vi "Device_Connect.vi"() -> ()   [LabVIEW 2020]
uses:
  User_Manage/User_Databse/User String.ctl
  <vilib>/Retry/UI Control Suite/Boolean/System Buttons/Connect Button.ctl
  Driver/E5071C/E5071C/E5071C.lvclass
  Driver/PEU/PEU/PEU.lvclass
  <vilib>/Utility/cursorutil.llb/Set Cursor (Icon Pict).vi
panel:
  in  "Title":string="设备连接"
  out "User Info":T1
  in  "Connect_PEU":T2
  in  "Port_PEU":u16=4001 caption="Port:"
  in  "IP_PEU":string="192.167.1.11" caption="IP Address:"
  out "Device_PEU":string caption="Device:"
  in  "Next Button":bool
  in  "Connect_E5071C":T2
  in  "Port_ENA":u16 caption="Port:"
  in  "IP_ENA":string="192.167.1.100" caption="IP Address:"
  out "Device_ENA":string caption="Device:"
  out "Time String":string
  # "E5071C"
  # "PEU"
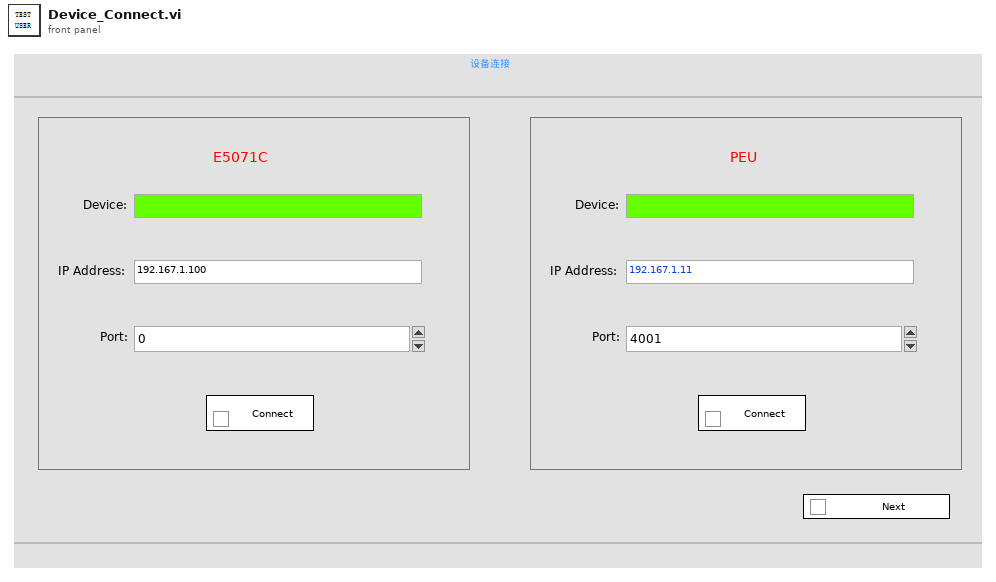
[diagram p1: front panel]
types:
  T1 = typedef "User String.ctl" = string
  T2 = typedef "Connect Button.ctl" = bool
  T3 = enum8{"Enabled", "Disabled", "Disabled and Grayed Out"}
  T4 = cluster{"User_Right":u16, "E5071C":refnum<class "E5071C.lvclass">, "PEU":refnum<class "PEU.lvclass">, "Next_OK":cluster{"ENA_OK":bool, "PEU_OK":bool}}
  T5 = typedef "User_Info.ctl" = cluster{"Name":string, "Password":string, "User_Right":u16, "Debuger?":bool, "Manager?":bool, "User_Remember_Name":bool, "User_Remember_PW":bool, "User_Right_String":string, "Null?":bool, "Language":string}
  T6 = enum32{"invalid app kind", "Development System", "Run Time System", "Student Edition", "Embedded LabVIEW", "Evaluation", "Custom"}
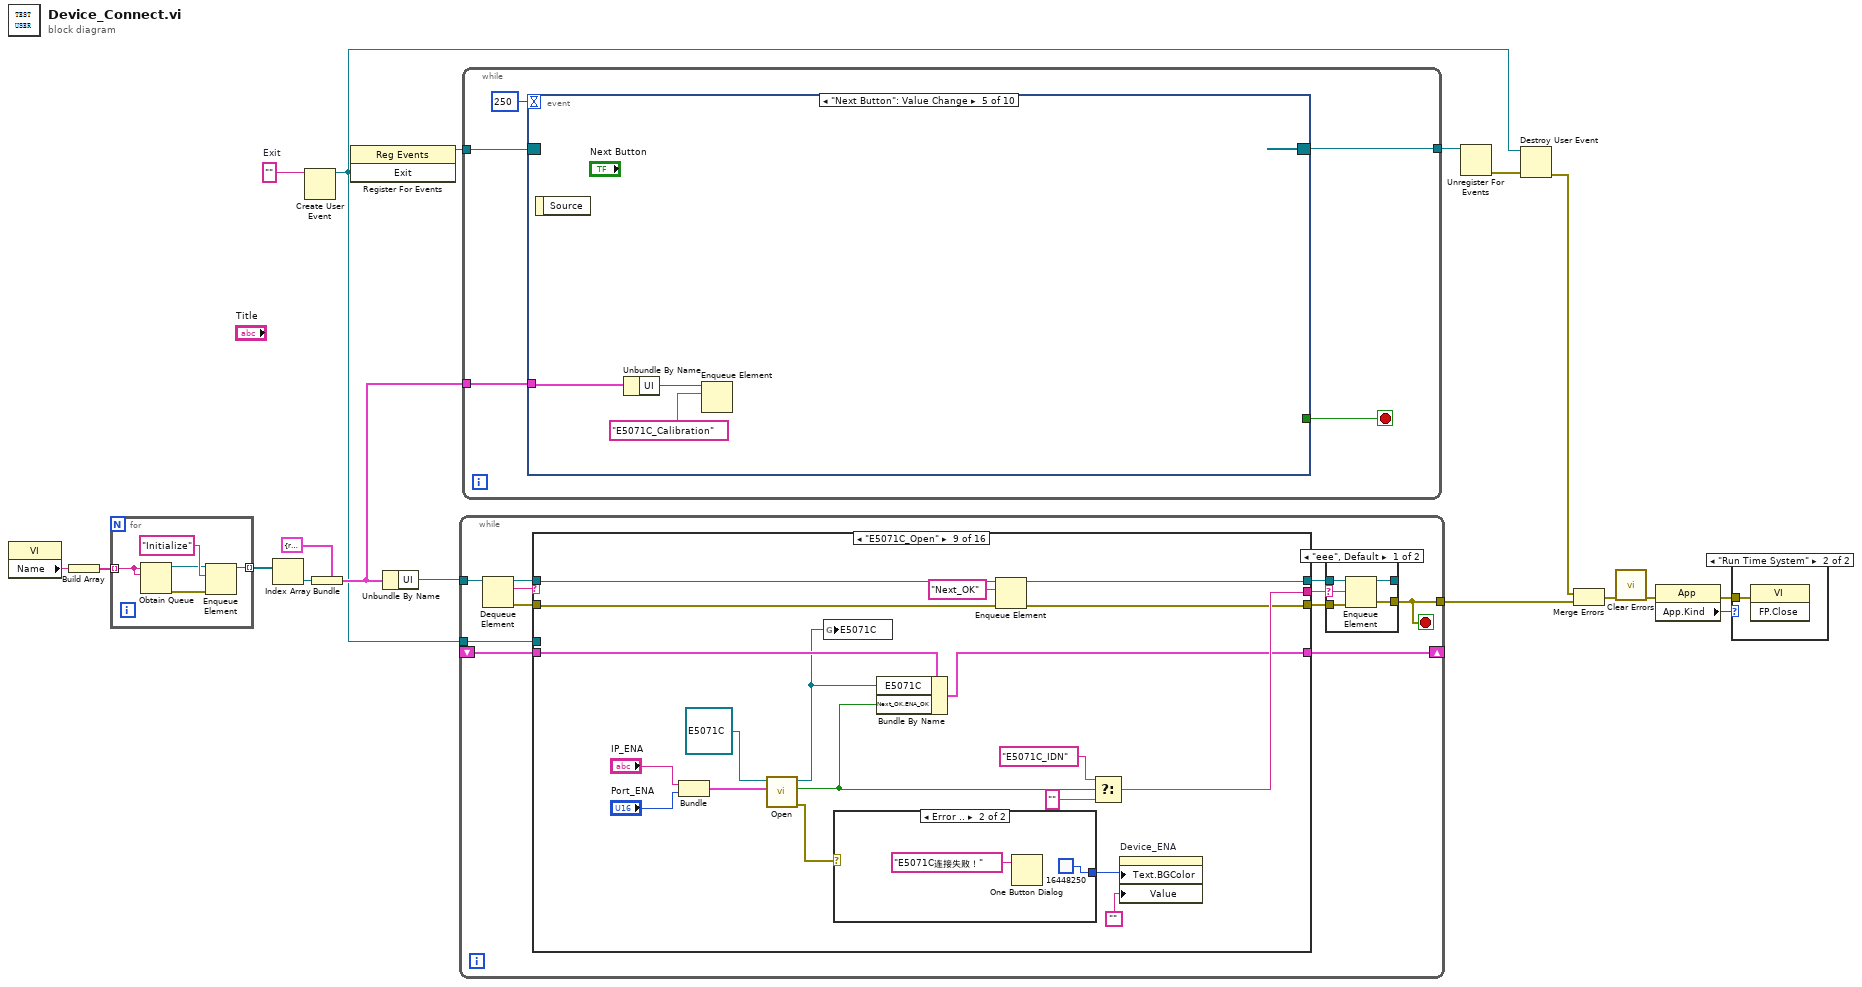
[diagram p0: block diagram]
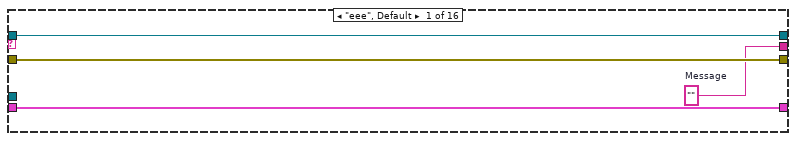
[diagram p4: hidden frame]
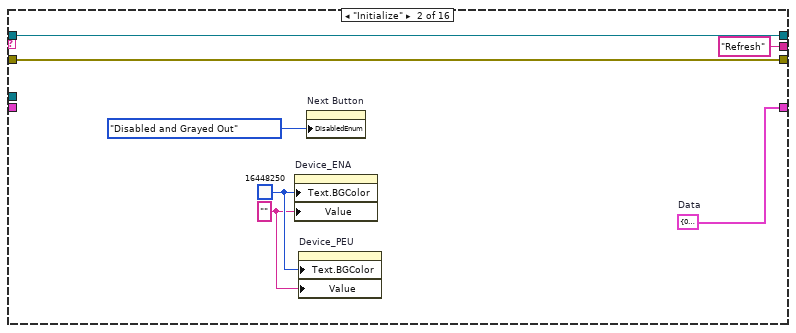
[diagram p5: hidden frame]
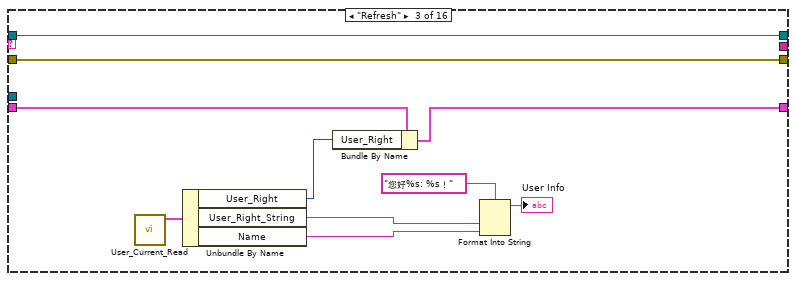
[diagram p6: hidden frame]
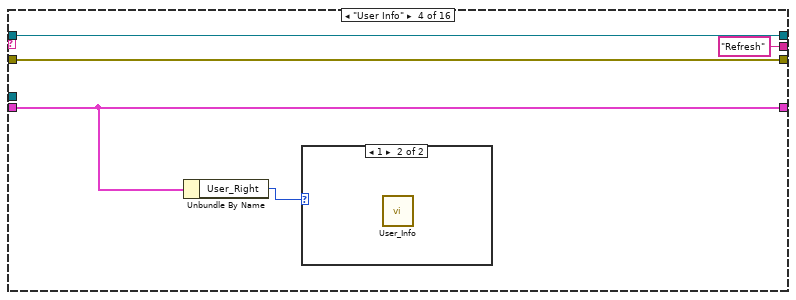
[diagram p7: hidden frame]
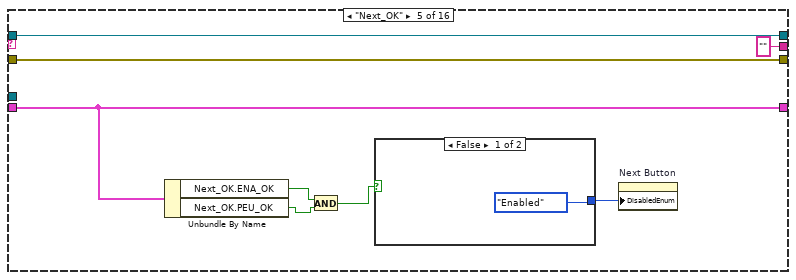
[diagram p9: hidden frame]
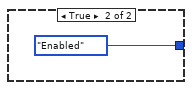
[diagram p10: hidden frame]
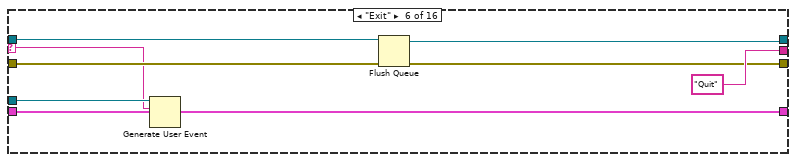
[diagram p11: hidden frame]
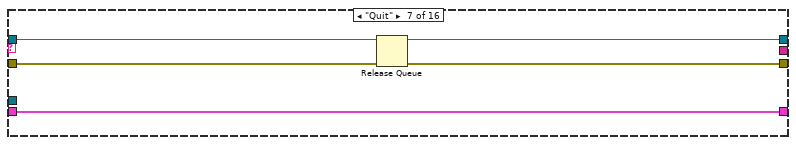
[diagram p12: hidden frame]
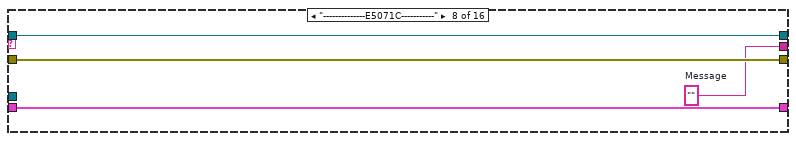
[diagram p13: hidden frame]
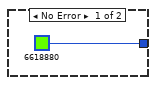
[diagram p14: hidden frame]
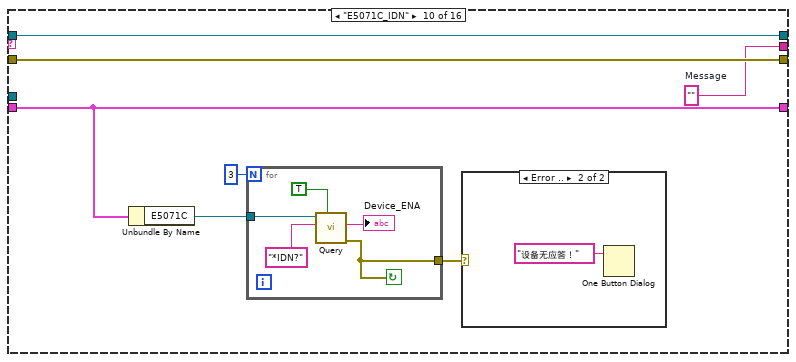
[diagram p15: hidden frame]
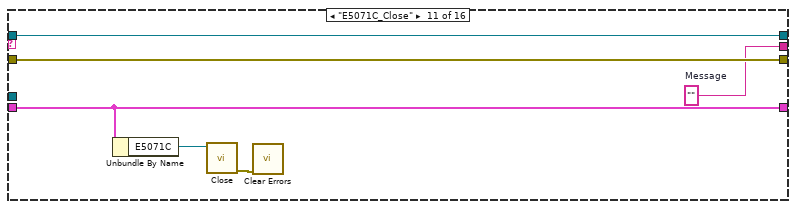
[diagram p17: hidden frame]
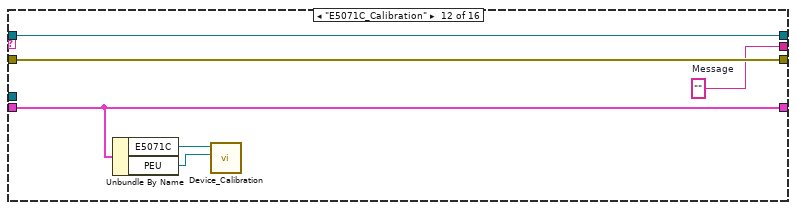
[diagram p18: hidden frame]
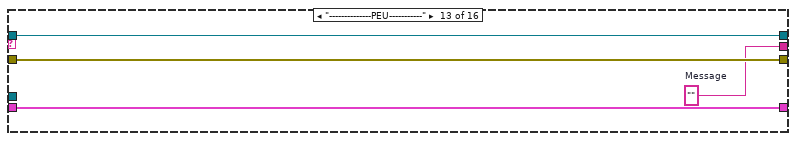
[diagram p19: hidden frame]
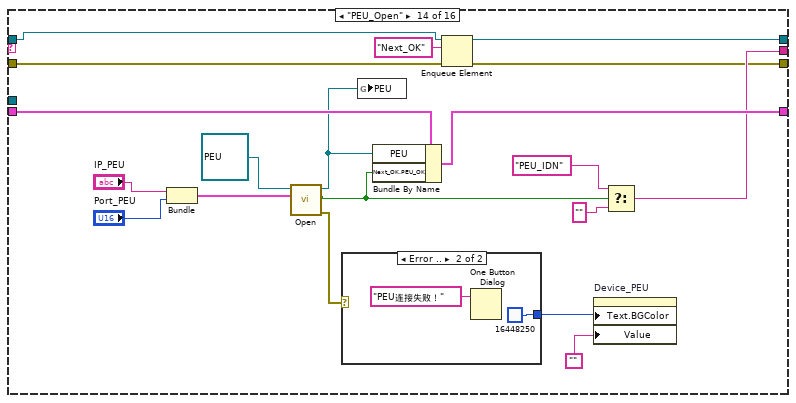
[diagram p20: hidden frame]
diagram:
  w3 = ""  # Exit
  n1 = property class="VI"() -> ("Name"=w13:string)  [unwired: 2 in, 2 out]
  n2 = Build Array(w13) -> (w14:string[])
  n3 = for {
    tunnel: w14 -> [w19] mode=indexing
    tunnel: [w20] -> w8 mode=indexing
    n4 = Obtain Queue(name (unnamed)=w19, element data type=w19) -> (queue out=w22:refnum<queue>, error out=w21:errorcluster)  [unwired: 3 in, 1 out]
    n5 = Enqueue Element(queue=w22, element="Initialize" ("元素"), error in (no error)=w21) -> (queue out=w20:refnum<queue>)  [unwired: 1 in, 2 out]
  }
  n6 = Index Array(array=w8) -> (element=w11:refnum<queue>)  [unwired: 1 in]
  n7 = Create User Event(user event datatype=w3) -> (user event=w7:refnum<user-event>)  [unwired: 1 in, 1 out]
  n8 = Bundle(cluster=cluster{"UI":refnum<queue>} {"UI"=refnum}, "UI"=w11) -> (w12:cluster{"UI":refnum<queue>})
  n9 = register-events(w7) -> (reference out=w4:refnum<event-registration>)  [unwired: 2 in, 1 out]
  n10 = Unbundle By Name(w12) -> ("UI"=w9:refnum<queue>)
  n11 = while {
    tunnel: w9 -> [w34]
    tunnel: [w24] -> w16
    shift-right: [w28] -> _
    shift-left: _ -> [w27]
    tunnel: w7 -> [w26]
    stop <- w24 stop-if-true
    n12 = Dequeue Element(queue=w34) -> (queue out=w33:refnum<queue>, element=w25:string, error out=w30:errorcluster)  [unwired: 2 in, 1 out]
    n13 = case shown="\"E5071C_Open\"" w25 {
      selector: w25 -> [_ _ _ _ _ w78 _ _ _ _ _ _ _ _ _ _]
      tunnel: w33 -> [w45 w52 w62 w67 w75 w83 w89 w93 w97 w122 w134 w140 w144 w147 w173 w185]
      tunnel: [w45 w52 w62 w67 w75 w82 w89 w93 w98 w122 w134 w140 w144 w146 w173 w185] -> w32
      tunnel: [w44 w51 w61 w66 w74 w81 w86 w92 w99 w121 w133 w139 w143 w149 w172 w184] -> w31
      tunnel: w30 -> [w44 w51 w61 w66 w74 w80 w88 w92 w100 w121 w133 w139 w143 w148 w172 w184]
      tunnel: [w43 "Refresh" ("Message") _ "Refresh" ("Message") "" ("Message") "Quit" ("Message") _ w91 w107 w120 w132 w138 w142 w152 w171 w183] -> w29
      tunnel: [w42 w50 w54 w64 w72 w85 w87 w90 w105 w119 w131 w137 w141 w158 w170 w182] -> w28
      tunnel: w27 -> [w42 _ w55 w64 w72 w85 w87 w90 w106 w119 w131 w137 w141 w159 w170 w182]
      tunnel: w26 -> [_ _ _ _ _ w79 _ _ _ _ _ _ _ _ _ _]
      frame "eee", Default {
        w43 = ""  # Message
      }
      frame "Initialize" {
        w47 = "" ("Device:")
        w48 = u32 16448250 ("Text.Text Colors:BG Color")
        w50 = T4 {"User_Right"=0, "E5071C"=refnum, "PEU"=refnum, "Next_OK"={"ENA_OK"=FALSE, "PEU_OK"=FALSE}}  # Data
        n14 = property on="Device_ENA" class="Str"("Text.BGColor"=w48, "Value"=w47) -> ()  [unwired: 2 in, 2 out]
        n15 = property on="Device_PEU" class="Str"("Text.BGColor"=w48, "Value"=w47) -> ()  [unwired: 2 in, 2 out]
        n16 = property on="Next Button" class="Bool"("DisabledEnum"=T3."Disabled and Grayed Out" ("Disabled")) -> ()  [unwired: 2 in, 2 out]
      }
      frame "Refresh" {
        n17 = call "User_Current_Read.vi"() -> ("User_Info"=w60:T5)  [unwired: 10 in, 1 out]
        n18 = Unbundle By Name(w60) -> ("User_Right"=w53:u16, "User_Right_String"=w59:string, "Name"=w58:string)
        n19 = Bundle By Name(cluster=w55, "User_Right"=w53) -> (w54:T4)
        n20 = Format Into String(format string="您好%s: %s！" ("格式字符串"), w59, w58) -> (resulting string=→"User Info":string)  [unwired: 2 in, 1 out]
      }
      frame "User Info" {
        n21 = Unbundle By Name(w64) -> ("User_Right"=w63:u16)
        n22 = case shown="1" w63 {
          frame 0, Default {
          }
          frame 1 {
            n23 = call "User_Info.vi"() -> ()  [unwired: 12 in]
          }
        }
      }
      frame "Next_OK" {
        n24 = Unbundle By Name(w72) -> ("Next_OK.ENA_OK"=w71:bool, "Next_OK.PEU_OK"=w70:bool)
        n25 = And(x=w71, y=w70) -> (x .and. y?=w68:bool)
        n26 = case shown="False" w68 {
          tunnel: [T3."Enabled" ("Disabled") T3."Enabled" ("Disabled")] -> w69
          frame False {
          }
          frame True {
          }
        }
        n27 = property on="Next Button" class="Bool"("DisabledEnum"=w69) -> ()  [unwired: 2 in, 2 out]
      }
      frame "Exit" {
        n28 = Generate User Event(user event=w79, event data cluster=w78) -> ()  [unwired: 2 in, 2 out]
        n29 = Flush Queue(queue=w83, error in (no error)=w80) -> (queue out=w82:refnum<queue>, error out=w81:errorcluster)  [unwired: 1 out]
      }
      frame "Quit" {
        n30 = Release Queue(queue=w89, error in (no error)=w88) -> (error out=w86:errorcluster)  [unwired: 1 in, 2 out]
      }
      frame "--------------E5071C-----------" {
        w91 = ""  # Message
      }
      frame "E5071C_Open" {
        n31 = Bundle("IP_ENA"="IP_ENA", "Port_ENA"="Port_ENA") -> (w110:cluster{"IP_ENA":string, "Port_ENA":u16})  [unwired: 1 in]
        n32 = call "Open.vi"("Link"=w110, "E5071C in"=refnum<class "E5071C.lvclass"> refnum ("E5071C.lvlib:E5071C.lvclass")) -> ("error out"=w95:errorcluster, "Link_OK"=w101:bool, "E5071C out"=w94:refnum<class "E5071C.lvclass">)  [unwired: 7 in]
        n33 = global write "Global.vi" "E5071C"(w94) -> ()
        n34 = case shown="Error .." w95 {
          tunnel: [u32 6618880 ("Text.Text Colors:BG Color") u32 16448250 ("Text.Text Colors:BG Color")] -> w103
          frame No Error {
          }
          frame Error {
            n35 = One Button Dialog(message="E5071C连接失败！") -> ()  [unwired: 1 in, 1 out]
          }
        }
        n36 = Bundle By Name(cluster=w106, "E5071C"=w94, "Next_OK.ENA_OK"=w101) -> (w105:T4)
        n37 = Enqueue Element(queue=w97, element="Next_OK", error in (no error)=w100) -> (queue out=w98:refnum<queue>, error out=w99:errorcluster)  [unwired: 1 in, 1 out]
        n38 = Select(t="E5071C_IDN", s=w101, f="") -> (s? t:f=w107:string)
        n39 = property on="Device_ENA" class="Str"("Text.BGColor"=w103, "Value"="") -> ()  [unwired: 2 in, 2 out]
      }
      frame "E5071C_IDN" {
        w120 = ""  # Message
        n40 = Unbundle By Name(w119) -> ("E5071C"=w118:refnum<class "E5071C.lvclass">)
        n41 = for {
          N: 3 -> [_]
          tunnel: w118 -> [w127]
          tunnel: [w124] -> w116
          stop <- w124 continue-if-true
          n42 = call "Query.vi"("Return"=TRUE, "Command"="*IDN?", "E5071C in"=w127) -> ("error out"=w124:errorcluster, "read buffer"=→"Device_ENA":string)  [unwired: 6 in, 1 out]
        }
        n43 = case shown="Error .." w116 {
          frame No Error {
          }
          frame Error {
            n44 = One Button Dialog(message="设备无应答！") -> ()  [unwired: 1 in, 1 out]
          }
        }
      }
      frame "E5071C_Close" {
        w132 = ""  # Message
        n45 = Unbundle By Name(w131) -> ("E5071C"=w130:refnum<class "E5071C.lvclass">)
        n46 = call "Close.vi"("E5071C in"=w130) -> ("error out"=w129:errorcluster)  [unwired: 9 in, 1 out]
        n47 = call <vilib>:"Clear Errors.vi"("error in (no error)"=w129) -> ()  [unwired: 5 in, 2 out]
      }
      frame "E5071C_Calibration" {
        w138 = ""  # Message
        n48 = Unbundle By Name(w137) -> ("E5071C"=w136:refnum<class "E5071C.lvclass">, "PEU"=w135:refnum<class "PEU.lvclass">)
        n49 = call "Device_Calibration.vi"("PEU"=w135, "E5071C"=w136) -> ()  [unwired: 10 in]
      }
      frame "--------------PEU-----------" {
        w142 = ""  # Message
      }
      frame "PEU_Open" {
        n50 = Bundle("IP_PEU"="IP_PEU", "Port_PEU"="Port_PEU") -> (w160:cluster{"IP_PEU":string, "Port_PEU":u16})  [unwired: 1 in]
        n51 = call "Open.vi"("Link"=w160, "PEU in"=refnum<class "PEU.lvclass"> refnum ("PEU.lvlib:PEU.lvclass")) -> ("error out"=w155:errorcluster, "Link_OK"=w151:bool, "PEU out"=w145:refnum<class "PEU.lvclass">)  [unwired: 7 in]
        n52 = case shown="Error .." w155 {
          tunnel: [u32 6618880 ("Text.Text Colors:BG Color") u32 16448250 ("Text.Text Colors:BG Color")] -> w153
          frame No Error {
          }
          frame Error {
            n53 = One Button Dialog(message="PEU连接失败！") -> ()  [unwired: 1 in, 1 out]
          }
        }
        n54 = global write "Global.vi" "PEU"(w145) -> ()
        n55 = Bundle By Name(cluster=w159, "PEU"=w145, "Next_OK.PEU_OK"=w151) -> (w158:T4)
        n56 = Enqueue Element(queue=w147, element="Next_OK", error in (no error)=w148) -> (queue out=w146:refnum<queue>, error out=w149:errorcluster)  [unwired: 1 in, 1 out]
        n57 = property on="Device_PEU" class="Str"("Text.BGColor"=w153, "Value"="") -> ()  [unwired: 2 in, 2 out]
        n58 = Select(t="PEU_IDN", s=w151, f="") -> (s? t:f=w152:string)
      }
      frame "PEU_IDN" {
        w171 = ""  # Message
        n59 = Unbundle By Name(w170) -> ("PEU"=w169:refnum<class "PEU.lvclass">)
        n60 = for {
          N: 3 -> [_]
          tunnel: w169 -> [w179]
          tunnel: [w176] -> w167
          stop <- w176 continue-if-true
          n61 = call "Query.vi"("Return"=TRUE, "Command"="*IDN?", "PEU in"=w179) -> ("error out"=w176:errorcluster, "read buffer"=→"Device_PEU":string)  [unwired: 6 in, 1 out]
        }
        n62 = case shown="Error .." w167 {
          frame No Error {
          }
          frame Error {
            n63 = One Button Dialog(message="设备无应答！") -> ()  [unwired: 1 in, 1 out]
          }
        }
      }
      frame "PEU_Close" {
        w183 = ""  # Message
        n64 = Unbundle By Name(w182) -> ("PEU"=w181:refnum<class "PEU.lvclass">)
        n65 = call "Close.vi"("PEU in"=w181) -> ("error out"=w180:errorcluster)  [unwired: 9 in, 1 out]
        n66 = call <vilib>:"Clear Errors.vi"("error in (no error)"=w180) -> ()  [unwired: 5 in, 2 out]
      }
    }
    n67 = case shown="\"eee\", Default" w29 {
      selector: w29 -> [w35 _]
      tunnel: w32 -> [w39 w41]
      tunnel: w31 -> [w38 w40]
      tunnel: [w37 w40] -> w24
      tunnel: [w36 w41] -> _
      frame "eee", Default {
        n68 = Enqueue Element(queue=w39, element=w35, error in (no error)=w38) -> (queue out=w36:refnum<queue>, error out=w37:errorcluster)  [unwired: 1 in, 1 out]
      }
      frame "" {
      }
    }
  }
  n69 = while {
    tunnel: w4 -> [w189]
    tunnel: [w188] -> w6
    tunnel: w12 -> [w187]
    stop <- w190 stop-if-true
    n70 = event shown="[4] \"Next Button\": Value Change" {
      selector: w189 -> [_ _ _ _ _ _ _ _ _ _]
      dyn-events: [_ _ _ _ _ _ _ _ _ _] -> w188
      timeout: 250 -> [_ _ _ _ _ _ _ _ _ _]
      tunnel: [_ _ _ _ _ w206 _ _ _ _] -> w190
      tunnel: w187 -> [_ _ w196 w199 w202 _ w210 w216 _ _]
      event Timeout {
        n71 = event-data() -> ()  [unwired: 1 in, 1 out]
        n72 = Format Date/Time String() -> (date/time string=→"Time String":string)  [unwired: 3 in]
      }
      event Key Down {
        n73 = event-data() -> ("Char"=w192:i16, "PlatMods.Ctrl"=w193:bool)  [unwired: 1 in]
        n74 = case shown="True" w193 {
          tunnel: w192 -> [_ w194]
          frame False {
          }
          frame True {
            n75 = case shown="101" w194 {
              frame 0, Default {
              }
              frame 101 {
                n76 = property class="VI"("BDWin.Open"=TRUE ("程序框图窗口:打开")) -> ()  [unwired: 2 in, 2 out]
              }
            }
          }
        }
      }
      event Value Change {
        n77 = event-data() -> ()  [unwired: 1 in, 1 out]
        n78 = Unbundle By Name(w196) -> ("UI"=w198:refnum<queue>)
        n79 = Enqueue Element(queue=w198, element="E5071C_Open" ("元素")) -> ()  [unwired: 2 in, 3 out]
      }
      event Value Change {
        n80 = event-data() -> ()  [unwired: 1 in, 1 out]
        n81 = Unbundle By Name(w199) -> ("UI"=w201:refnum<queue>)
        n82 = Enqueue Element(queue=w201, element="PEU_Open" ("元素")) -> ()  [unwired: 2 in, 3 out]
      }
      event "Next Button": Value Change {
        n83 = event-data() -> ()  [unwired: 1 in, 1 out]
        n84 = Unbundle By Name(w202) -> ("UI"=w204:refnum<queue>)
        n85 = Enqueue Element(queue=w204, element="E5071C_Calibration" ("元素")) -> ()  [unwired: 2 in, 3 out]
      }
      event User Event {
        n86 = event-data() -> ("Exit"=w207:string)  [unwired: 1 in]
        n87 = Equal?(x=w207, y="Exit") -> (x = y?=w206:bool)
      }
      event Panel Close? {
        n88 = event-data() -> ()  [unwired: 1 in, 1 out]
        n89 = Cluster To Array(cluster=w210) -> (array=w209:refnum<queue>[])
        n90 = for {
          tunnel: w209 -> [w213] mode=indexing
          tunnel: "Exit" ("元素") -> [w212]
          n91 = Enqueue Element(queue=w213, element=w212) -> ()  [unwired: 2 in, 3 out]
        }
        n92 = event-data("Discard?"=TRUE ("放弃？")) -> ()  [unwired: 1 in, 1 out]
      }
      event Mouse Down {
        n93 = event-data() -> ()  [unwired: 1 in, 1 out]
        n94 = Unbundle By Name(w216) -> ("UI"=w215:refnum<queue>)
        n95 = Enqueue Element(queue=w215, element="User Info" ("元素")) -> ()  [unwired: 2 in, 3 out]
      }
      event Mouse Enter {
        n96 = event-data() -> ()  [unwired: 1 in, 4 out]
        n97 = call-poly <vilib>:"Set Cursor.vi"("icon"=u16 6) -> ()  [unwired: 9 in, 2 out]
      }
      event Mouse Leave {
        n98 = event-data() -> ()  [unwired: 1 in, 4 out]
        n99 = call-poly <vilib>:"Set Cursor.vi"("icon"=u16 0) -> ()  [unwired: 9 in, 2 out]
      }
    }
  }
  n100 = Unregister For Events(event registration refnum=w6) -> (error out=w5:errorcluster)  [unwired: 1 in]
  n101 = Destroy User Event(user event=w7, error in=w5) -> (error out=w15:errorcluster)
  n102 = Merge Errors(w15, w16) -> (w17:errorcluster)
  n103 = call <vilib>:"Clear Errors.vi"("error in (no error)"=w17) -> ("error out"=w18:errorcluster)  [unwired: 5 in, 1 out]
  n104 = property class="App"(error in=w18) -> (error out=w1:errorcluster, "App.Kind"=w2:T6)  [unwired: 1 in, 1 out]
  n105 = case shown="\"Run Time System\"" w2 {
    tunnel: w1 -> [_ w219]
    frame "invalid app kind", Default {
    }
    frame "Run Time System" {
      n106 = invoke class="VI" method="FP.Close"(error in=w219) -> ()  [unwired: 2 in, 3 out]
    }
  }
